vi "Parse MISSION_ACK.vi"(11 "Data":string) -> (3 "Mission Acknowledge":T1)   [LabVIEW 2014]
uses:
  Controls/Mission Planning Controls/MAVLink Mission Ack.ctl
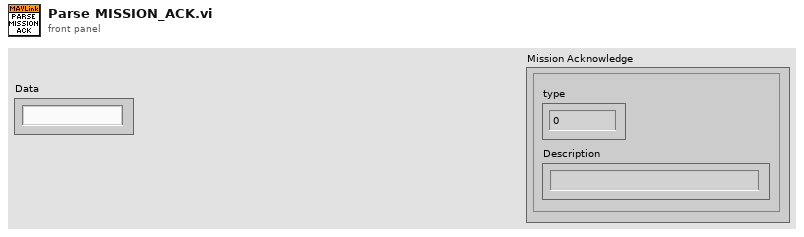
[diagram p1: front panel]
types:
  T1 = typedef "MAVLink Mission Ack.ctl" = cluster{"type":u8, "Description":string}
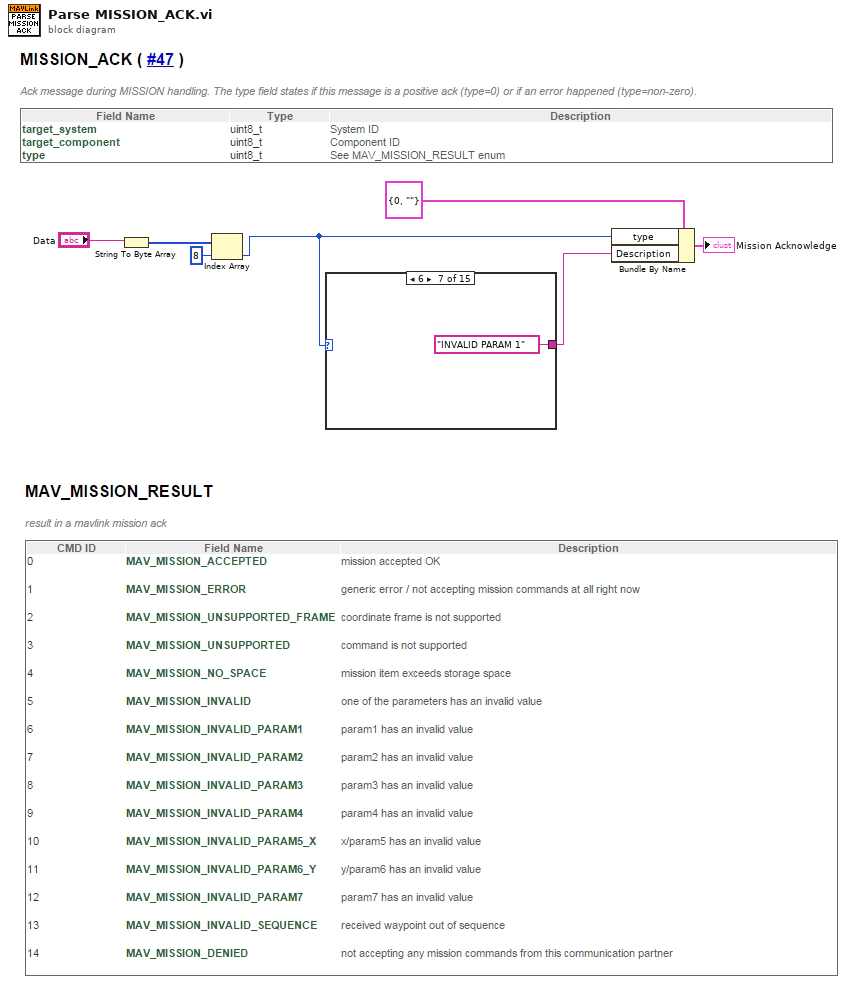
[diagram p0: block diagram]
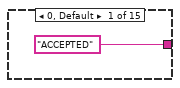
[diagram p2: hidden frame]
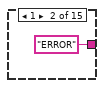
[diagram p3: hidden frame]
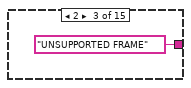
[diagram p4: hidden frame]
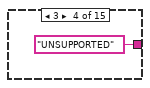
[diagram p5: hidden frame]
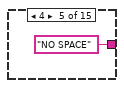
[diagram p6: hidden frame]
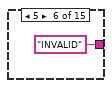
[diagram p7: hidden frame]
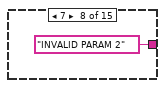
[diagram p8: hidden frame]
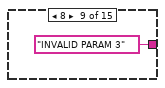
[diagram p9: hidden frame]
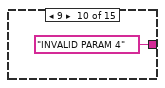
[diagram p10: hidden frame]
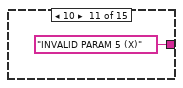
[diagram p11: hidden frame]
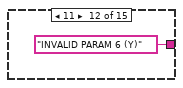
[diagram p12: hidden frame]
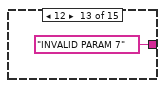
[diagram p13: hidden frame]
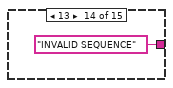
[diagram p14: hidden frame]
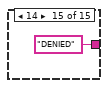
[diagram p15: hidden frame]
diagram:
  n1 = String To Byte Array(string="Data") -> (unsigned byte array=w6:u8[])
  n2 = Index Array(array=w6, index=8) -> (element=w3:u8)
  n3 = case shown="6" w3 {
    tunnel: ["ACCEPTED" "ERROR" "UNSUPPORTED FRAME" "UNSUPPORTED" "NO SPACE" "INVALID" "INVALID PARAM 1" "INVALID PARAM 2" "INVALID PARAM 3" "INVALID PARAM 4" "INVALID PARAM 5 (X)" "INVALID PARAM 6 (Y)" "INVALID PARAM 7" "INVALID SEQUENCE" "DENIED"] -> w2
    frame 0, Default {
    }
    frame 1 {
    }
    frame 2 {
    }
    frame 3 {
    }
    frame 4 {
    }
    frame 5 {
    }
    frame 6 {
    }
    frame 7 {
    }
    frame 8 {
    }
    frame 9 {
    }
    frame 10 {
    }
    frame 11 {
    }
    frame 12 {
    }
    frame 13 {
    }
    frame 14 {
    }
  }
  n4 = Bundle By Name(cluster=T1 {"type"=0, "Description"=""} ("Mission Acknowledge"), "type"=w3, "Description"=w2) -> (→"Mission Acknowledge":T1)
